vi "Build.vi"(6 "Build":bool[](array[boolean]), 8 "error in (no error)":errorcluster, 9 "Pre-Release (None)":string, 10 "Version":T1, 11 "Builder in":refnum<class "Builder.lvclass">) -> (0 "error out":errorcluster, 3 "Builder out":refnum<class "Builder.lvclass">)   [LabVIEW 2020, in "Builder Tools.lvlib" / "Builder.lvclass"]
uses:
  Builder.lvclass
  Builder Core/Version.ctl
  Builder.lvclass/Builder.ctl
  Build Async.vi
  Builder Core/Builder Core.lvlib
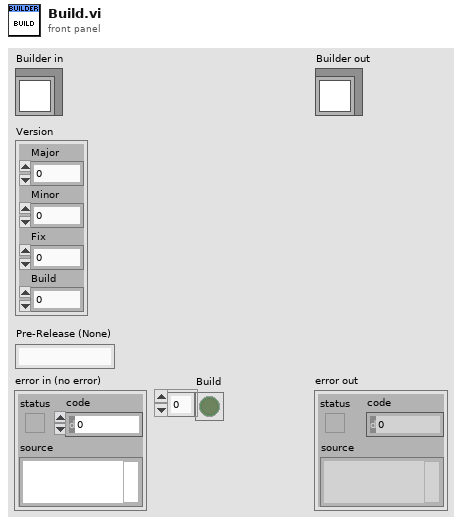
[diagram p1: front panel]
types:
  T1 = typedef "Builder Core.lvlib/Version.ctl" = cluster{"Major":u16, "Minor":u16, "Fix":u16, "Build":u16}
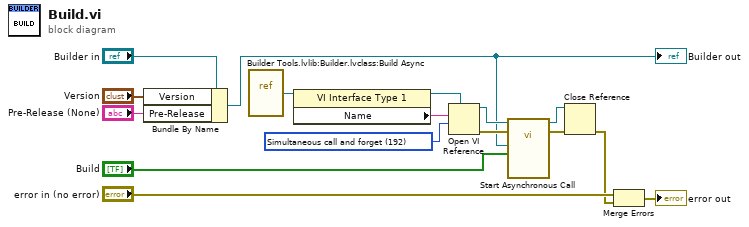
[diagram p0: block diagram]
diagram:
  w10 = 192 items=["Record modifications"=1, "Open templates for editing"=2, "Prompt user to save"=4, "Prepare for reentrant run"=8, "Prompt to find missing subVIs"=16, "Hide loading dialog box"=32, "Enable simultaneous calls"=64, "Prepare to call and forget"=128, "Simultaneous call and forget"=192, "Prepare to call and collect"=256, "Simultaneous call and collect"=320]
  n1 = Bundle By Name(cluster="Builder in", "Version"="Version", "Pre-Release"="Pre-Release (None)") -> (w4:refnum<class "Builder.lvclass">)
  "Builder out" <- w4
  n2 = vi-ref "Builder Tools.lvlib:Builder.lvclass:Build Async.vi"() -> (w8:refnum<vi>)
  n3 = property class="VI Interface Type 1"(reference=w8) -> (reference out=w11:refnum<vi>, "Name"=w9:string)  [unwired: 1 in, 1 out]
  n4 = Open VI Reference(type specifier VI Refnum (for type only)=w11, vi path=w9, options=w10) -> (vi reference=w13:refnum<vi>, error out=w12:errorcluster)  [unwired: 3 in]
  n5 = call-by-ref "Start Asynchronous Call"(reference=w13, error in=w12, "Build"="Build", "Builder in"=w4) -> (reference out=w15:refnum<vi>, error out=w14:errorcluster)  [unwired: 10 in]
  n6 = Close Reference(reference=w15, error in (no error)=w14) -> (error out=w6:errorcluster)
  n7 = Merge Errors("error in (no error)", w6) -> (→"error out":errorcluster)
